vi "Fit Scale Range to Content.vi"(11 "Base Graph in":refnum<class "Base Graph.lvclass">) -> (3 "Base Graph out":refnum<class "Base Graph.lvclass">)   [LabVIEW 2023, in "Base Graph.lvclass"]
uses:
  Base Graph.lvclass
  Base Graph.lvclass/Base Graph.ctl
panel:
  # "PREVENTS AFTER DEZOOMING THE INTENSITY GRAPH IS 1PIXEL TO WIDE"
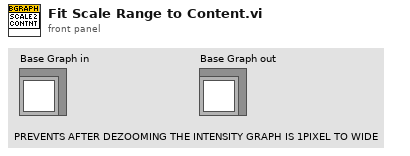
[diagram p1: front panel]
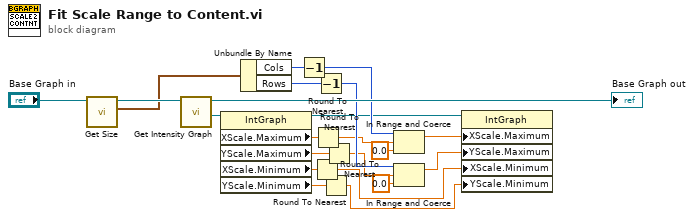
[diagram p0: block diagram]
diagram:
  n1 = call "Get Size.vi"("Base Graph in"="Base Graph in") -> ("Size"=w18:cluster{"Rows":u32, "Cols":u32}, "Base Graph out"=w20:refnum<class "Base Graph.lvclass">)  [unwired: 9 in]
  n2 = call "Get Intensity Graph.vi"("Base Graph in"=w20) -> ("Intensity Graph"=w19:refnum<vi>, "Base Graph out"=→"Base Graph out":refnum<class "Base Graph.lvclass">)  [unwired: 9 in]
  n3 = property class="IntGraph"(reference=w19) -> (reference out=w9:refnum<vi>, "XScale.Maximum"=w17:dbl, "YScale.Maximum"=w13:dbl, "XScale.Minimum"=w6:dbl, "YScale.Minimum"=w5:dbl)  [unwired: 1 in, 1 out]
  n4 = Unbundle By Name(w18) -> ("Cols"=w16:u32, "Rows"=w12:u32)
  n5 = Decrement(x=w16) -> (x-1=w15:u32)
  n6 = Round To Nearest(number=w6) -> (nearest integer value=w2:dbl)
  n7 = Round To Nearest(number=w17) -> (nearest integer value=w4:dbl)
  n8 = Decrement(x=w12) -> (x-1=w11:u32)
  n9 = Round To Nearest(number=w5) -> (nearest integer value=w1:dbl)
  n10 = Round To Nearest(number=w13) -> (nearest integer value=w3:dbl)
  n11 = In Range and Coerce(upper limit=w15, x=w4, lower limit=0.0) -> (coerced(x)=w8:dbl)  [unwired: 1 out]
  n12 = In Range and Coerce(upper limit=w11, x=w3, lower limit=0.0) -> (coerced(x)=w7:dbl)  [unwired: 1 out]
  n13 = property class="IntGraph"(reference=w9, "XScale.Maximum"=w8, "YScale.Maximum"=w7, "XScale.Minimum"=w2, "YScale.Minimum"=w1) -> ()  [unwired: 1 in, 2 out]
